vi "Lookup Command.vi"(0 "UART_Command in":T1, 5 "Baud":u32) -> (4 "UART_Command out":T1, 6 "Numeric":u16)   [LabVIEW 2012, in "UART_Host_Driver.lvlib" / "UART Driver.lvclass"]
uses:
  UART Driver.lvclass
  FPGA/UART/UART_Command.ctl
  FPGA/UART/UART_Firmware.lvlib
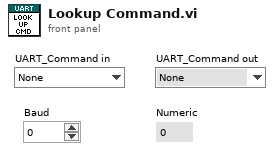
[diagram p1: front panel]
types:
  T1 = typedef "UART_Firmware.lvlib/UART_Command.ctl" = enum8{"None", "Tx", "SetBaud_High", "SetBaud_Low", "SetCharLength", "SetParity", "SetStopBits", "SetSpacing_High", "SetSpacing_Low"}
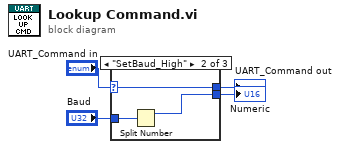
[diagram p0: block diagram]
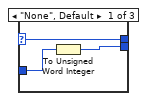
[diagram p2: hidden frame]
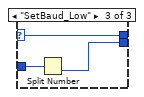
[diagram p3: hidden frame]
diagram:
  n1 = case shown="\"SetBaud_High\"" "UART_Command in" {
    selector: "UART_Command in" -> [w7 w10 w13]
    tunnel: [w7 w10 w13] -> w2
    tunnel: "Baud" -> [w6 w9 w12]
    tunnel: [w5 w8 w11] -> w3
    frame "None", Default {
      n2 = To Unsigned Word Integer(number=w6) -> (unsigned 16bit integer=w5:u16)
    }
    frame "SetBaud_High" {
      n3 = Split Number(x=w9) -> (hi(x)=w8:u16)  [unwired: 1 out]
    }
    frame "SetBaud_Low" {
      n4 = Split Number(x=w12) -> (lo(x)=w11:u16)  [unwired: 1 out]
    }
  }
  "Numeric" <- w3
  "UART_Command out" <- w2
